vi "XYZ to Angles.vi"(9 "Z Target Position":dbl, 10 "Y Target Position":dbl, 11 "X Target Position":dbl) -> (1 "Elbow Angle":dbl, 2 "Shoulder Angle":dbl, 3 "Turret Angle":dbl)   [LabVIEW 2018]
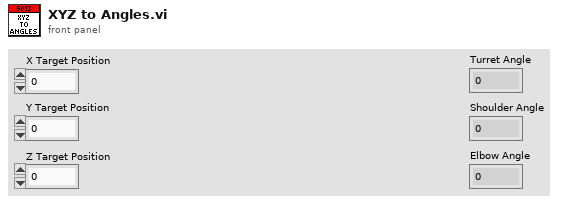
[diagram p1: front panel]
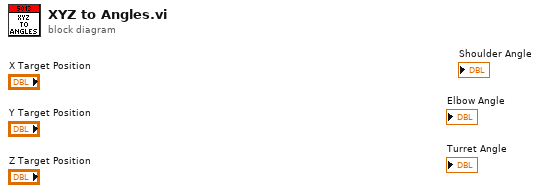
[diagram p0: block diagram]
diagram:
